vi "Get ID.vi"(10 "id":i32, 11 "devNum":i32) -> (2 "id out":i32, 3 "function return":u32)   [LabVIEW 2018, in "AndorSDK.lvlib"]
doc: "EXPNETTYPE unsigned int WINAPI GetID(int devNum, int * id);"
uses:
  AndorSDK.lvlib
  ATMCD32D.dll
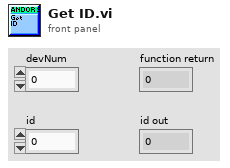
[diagram p1: front panel]
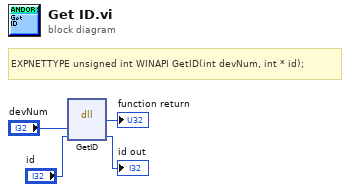
[diagram p0: block diagram]
diagram:
  # "EXPNETTYPE unsigned int WINAPI GetID(int devNum, int * id);"
  n1 = dll-call lib="PTH2babs E\nPersönliches02 - Arbeit03-HiwijobsLabviewCodelibANDOR\tAndor SDK\nATMCD32D.*" fn="GetID"("devNum"="devNum", "id"="id") -> (→"function return":u32, "id"=→"id out":i32)  [unwired: 4 in, 2 out]
